vi "9_1_recursiveSearch.vi"(9 "key":i32, 10 "Map":map{i32, i32[]}(c390), 11 "In":i32[](array[numeric])) -> (3 "New Value":i32)   [LabVIEW 2021, in "2023.lvlib"]
uses:
  2023.lvlib
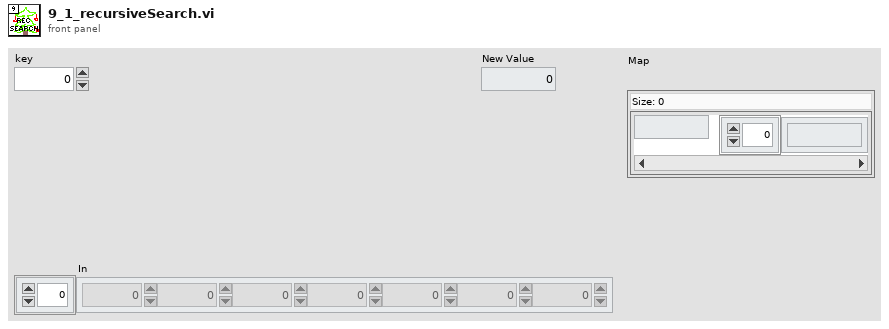
[diagram p1: front panel]
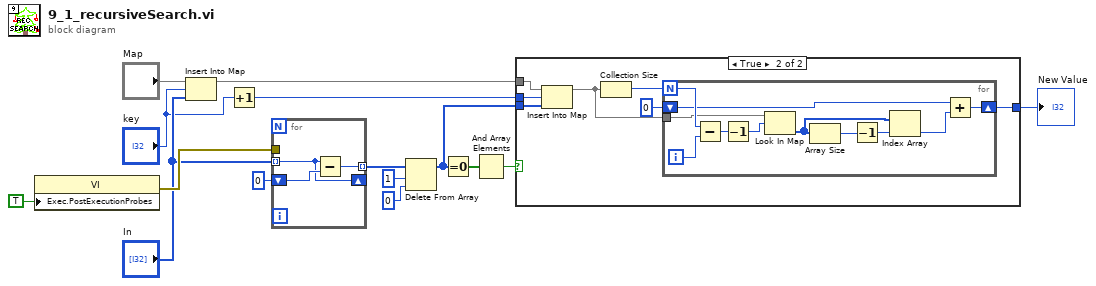
[diagram p0: block diagram]
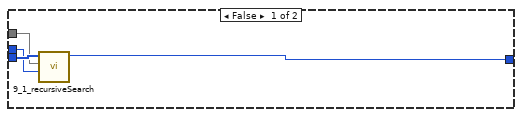
[diagram p2: hidden frame]
diagram:
  n1 = property class="VI"("Exec.PostExecutionProbes"=TRUE ("Execution:Retain Wire Values")) -> (error out=w8:errorcluster)  [unwired: 2 in, 1 out]
  n2 = Insert Into Map(map in="Map", key="key", value="In") -> (map out=w5:map{i32, i32[]})  [unwired: 2 out]
  n3 = Increment(x="key") -> (x+1=w2:i32)
  n4 = for {
    shift-right: [w16] -> _
    shift-left: 0 -> [w18]
    tunnel: [w17] -> w14 mode=indexing
    tunnel: "In" -> [w16] mode=indexing
    tunnel: w8 -> [_]
    n5 = Subtract(x=w16, y=w18) -> (x-y=w17:i32)
  }
  n6 = Delete From Array(array=w14, length=1, index=0) -> (array with subset deleted=w7:i32[])  [unwired: 1 out]
  n7 = Equal To 0?(x=w7) -> (x = 0?=w11:bool[])
  n8 = And Array Elements(Boolean array=w11) -> (logical AND=w10:bool)
  n9 = case shown="True" w10 {
    tunnel: w7 -> [w22 w23]
    tunnel: w5 -> [w21 w26]
    tunnel: w2 -> [w20 w24]
    tunnel: [w19 w27] -> w1
    frame False {
      n10 = call "9_1_recursiveSearch.vi"("key"=w20, "Map"=w21, "In"=w22) -> ("New Value"=w19:i32)  [unwired: 8 in]
    }
    frame True {
      n11 = Insert Into Map(map in=w26, key=w24, value=w23) -> (map out=w25:map{i32, i32[]})  [unwired: 2 out]
      n12 = Collection Size(1:w25) -> (0:w29:i32)
      n13 = for {
        N: w29 -> [w40]
        tunnel: w25 -> [w39]
        shift-right: [w32] -> w27
        shift-left: 0 -> [w31]
        i -> [w38]
        n14 = Subtract(x=w40, y=w38) -> (x-y=w37:i32)
        n15 = Decrement(x=w37) -> (x-1=w36:i32)
        n16 = Look In Map(map=w39, key=w36) -> (value=w35:i32[])  [unwired: 1 in, 1 out]
        n17 = Array Size(array=w35) -> (size(s)=w34:i32)
        n18 = Decrement(x=w34) -> (x-1=w30:i32)
        n19 = Index Array(array=w35, index=w30) -> (element=w33:i32)
        n20 = Add(x=w31, y=w33) -> (x+y=w32:i32)
      }
    }
  }
  "New Value" <- w1
